vi "Analog Input.vi"() -> ()   [LabVIEW 2015]
doc: "Analog Input Example\n\nThis example will read voltages from an analog channel and display it on a chart. It will also display the average voltage over time. \n\nThe values for Average Bits and Samples Per Second on the front panel can be set while the VI is running.\n\nThis example expects a USB cable connected from your development PC to the Type B USB Jack (next to the power input) on the roboRIO."
uses:
  <vilib>/Rock Robotics/SystemInterfaces/AI/FPGA_AIChannel.ctl
  <vilib>/Rock Robotics/WPI/MotorControl/WPI_MotorControlDeviceRef.ctl
  <vilib>/Rock Robotics/WPI/MotorControl/WPI_MotorControlType.ctl
  <vilib>/Rock Robotics/SystemInterfaces/DIO/FPGA_DIOPWMChannel.ctl
  <vilib>/Rock Robotics/WPI/PWM/WPI_PWMDeadband.ctl
  <vilib>/Rock Robotics/WPI/CAN/Jaguar/SubVIs/WPI_CANJaguar_ControlMode.ctl
  <vilib>/Rock Robotics/WPI/CAN/TalonSRX/WPI_CANTalonSRX_APIControlMode.ctl
  <vilib>/Rock Robotics/WPI/MotorControl/WPI_MotorControlOpen Victor.vi
panel:
  out "MotorControlDevRef":T1={"DeviceStatus"={"status"=FALSE, "code"=0, "source"=""}, "Type"=enum."PWM", "PWM"={"PWM Channel"=enum."Invalid", "DeadBand"={"Name"="", "maxPositivePwm"=0, "minPositivePwm"=0, "centerPwm"=0, "maxNegativePwm"=0, "minNegativePwm"=0, "angularRange"=0}}, "CAN"={"Device Number"=0, "Control Mode"=enum."Percent VBus", "Semaphore"=refnum, "Max Vout"=12.0, "TalonSRX Control Mode"=enum."Percent VBus"}, "Invert"=FALSE}
  out "error out":errorcluster
  out "Motor Output":dbl
  in  "Output":dbl(slide) scale=-1.0..1.0
  in  "Samples Per Second":dbl=1000.0
  in  "Average Bits":u8=3 max=15
  in  "Channel":T8=enum."AI 2"
  out "Voltage Display":cluster{"Value":dbl, "Voltage":dbl}(graph)
  out "Average Voltage":dbl
  out "Voltage":dbl
  in  "stop":bool
  # "Set this input before running."
  # "These can be set while running."
  # "This chart displays the voltage and average voltage over time."
  # "This shows wiring for a typical analog input using a potentiometer.  In this case the potentiometer is being powered with 5 volts, and the Signal returned will vary from 0 to 5 volts"
  # "potentiometer"
  # "Gnd"
  # "S"
  # "V"
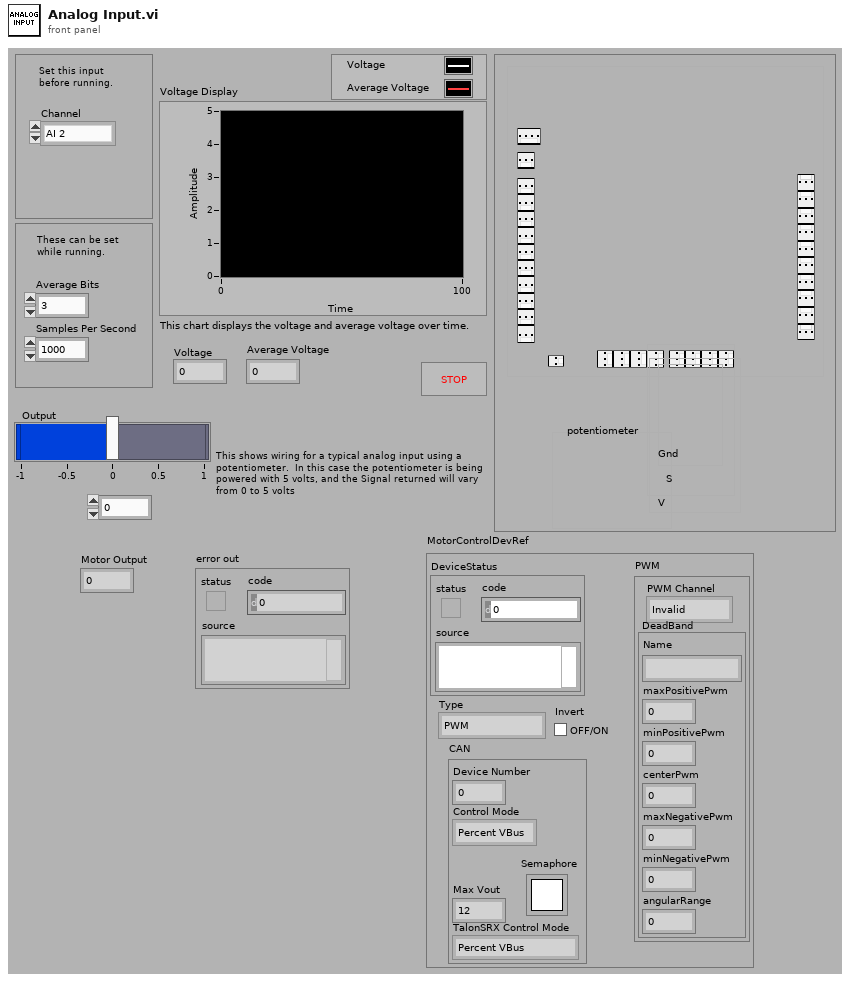
[diagram p1: front panel]
types:
  T1 = typedef "WPI_MotorControlDeviceRef.ctl" = cluster{"DeviceStatus":errorcluster, "Type":T2, "PWM":cluster{"PWM Channel":T3, "DeadBand":T4}, "CAN":cluster{"Device Number":u8, "Control Mode":T5, "Semaphore":T6, "Max Vout":dbl, "TalonSRX Control Mode":T7}, "Invert":bool}
  T2 = typedef "WPI_MotorControlType.ctl" = enum16{"PWM", "CAN", "CANTalonSRX"}
  T3 = typedef "FPGA_DIOPWMChannel.ctl" = enum8{"PWM 0", "PWM 1", "PWM 2", "PWM 3", "PWM 4", "PWM 5", "PWM 6", "PWM 7", "PWM 8", "PWM 9", "PWM MXP 0", "PWM MXP 1", "PWM MXP 2", "PWM MXP 3", "PWM MXP 4", "PWM MXP 5", "PWM MXP 6", "PWM MXP 7", "PWM MXP 8", "PWM MXP 9", "Invalid"}
  T4 = typedef "WPI_PWMDeadband.ctl" = cluster{"Name":string, "maxPositivePwm":i32, "minPositivePwm":i32, "centerPwm":i32, "maxNegativePwm":i32, "minNegativePwm":i32, "angularRange":u16}
  T5 = typedef "WPI_CANJaguar_ControlMode.ctl" = enum8{"Percent VBus", "Current", "Speed", "Position", "Voltage"}
  T6 = typedef "Semaphore RefNum" = refnum<k1>
  T7 = typedef "WPI_CANTalonSRX_APIControlMode.ctl" = enum8{"Percent VBus", "Speed", "Position", "Slave", "Unchanged / Invalid", "Voltage Compensation", "Current", "Motion Profile"}
  T8 = typedef "FPGA_AIChannel.ctl" = enum8{"AI 0", "AI 1", "AI 2", "AI 3", "AI MXP 0", "AI MXP 1", "AI MXP 2", "AI MXP 3", "Invalid"}
  T9 = typedef "WPI_AnalogChannelDevRef.ctl" = cluster{"DevStatus":errorcluster, "Analog Channel":T8}
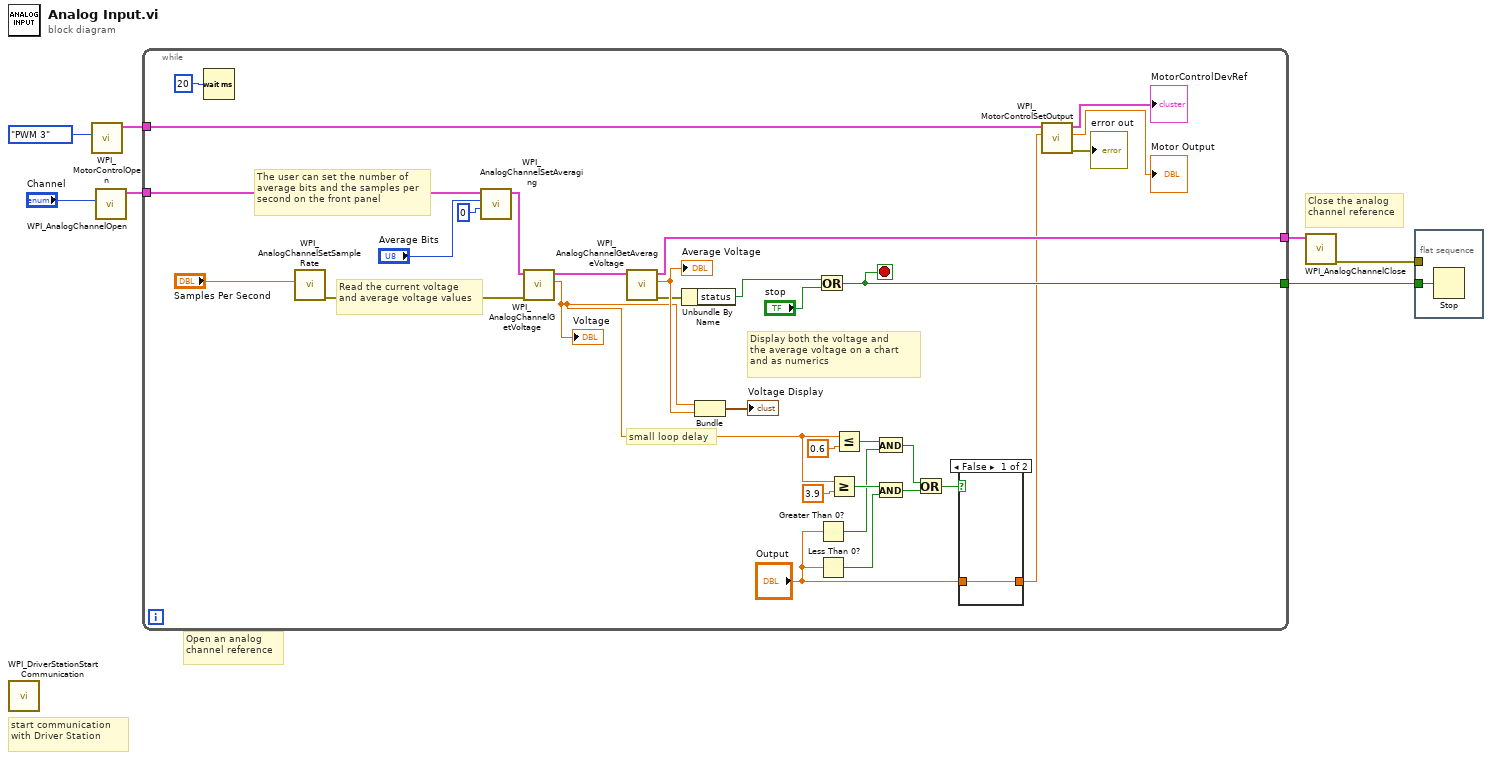
[diagram p0: block diagram]
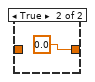
[diagram p2: hidden frame]
diagram:
  # "start communication with Driver Station"
  # "Close the analog\nchannel reference"
  # "Open an analog channel reference"
  n1 = call <vilib>:"WPI_DriverStationStart Communication.vi"() -> ()  [unwired: 2 in, 10 out]
  n2 = call-poly <vilib>:"WPI_MotorControlOpen.vi"("PWM Channel"=FPGA_DIOPWMChannel."PWM 3") -> ("MotorControlDeviceRef"=w1:T1)  [unwired: 9 in, 1 out]
  n3 = call <vilib>:"WPI_AnalogChannelOpen.vi"("Analog Channel"="Channel") -> ("AIDeviceRef"=w7:T9)  [unwired: 2 in, 8 out]
  n4 = while {
    tunnel: w7 -> [w33]
    tunnel: [w37] -> w6
    tunnel: [w24] -> w4
    tunnel: w1 -> [w23]
    stop <- w24 stop-if-true
    # "small loop delay"
    # "Read the current voltage\nand average voltage values"
    # "Display both the voltage and\nthe average voltage on a chart\nand as numerics"
    # "The user can set the number of \naverage bits and the samples per\nsecond on the front panel"
    n5 = Wait (ms)(milliseconds to wait=u32 20) -> ()  [unwired: 1 out]
    n6 = call <vilib>:"WPI_AnalogChannelSetSampleRate.vi"("Samples Per Second (per channel)"="Samples Per Second") -> ("error out"=w25:errorcluster)  [unwired: 4 in, 6 out]
    n7 = call <vilib>:"WPI_AnalogChannelSetAveraging.vi"("OversampleBits"=u8 0, "AverageBits"="Average Bits", "AIDeviceRef"=w33) -> ("AIDeviceRef"=w27:T9)  [unwired: 1 in, 7 out]
    n8 = call <vilib>:"WPI_AnalogChannelGetVoltage.vi"("error in (no error)"=w25, "AIDeviceRef"=w27) -> ("Voltage"=w12:dbl, "AIDeviceRef"=w38:T9)  [unwired: 8 out]
    "Voltage" <- w12
    n9 = call <vilib>:"WPI_AnalogChannelGetAverageVoltage.vi"("AIDeviceRef"=w38) -> ("error out"=w26:errorcluster, "Voltage"=w36:dbl, "AIDeviceRef"=w37:T9)  [unwired: 1 in, 7 out]
    "Average Voltage" <- w36
    n10 = Unbundle By Name(w26) -> ("status"=w31:bool)
    n11 = Bundle("Voltage"=w12, "Voltage"=w36) -> (→"Voltage Display":cluster{"Voltage":dbl, "Voltage":dbl})  [unwired: 1 out]
    n12 = Or(x=w31, y="stop") -> (x .or. y?=w24:bool)
    n13 = Greater Than 0?(x="Output") -> (x > 0?=w9:bool)
    n14 = Less Than 0?(x="Output") -> (x < 0?=w17:bool)
    n15 = Greater Or Equal?(x=w12, y=3.9) -> (x >= y?=w16:bool)
    n16 = Less Or Equal?(x=w12, y=0.6) -> (x <= y?=w11:bool)
    n17 = And(x=w11, y=w9) -> (x .and. y?=w8:bool)
    n18 = And(x=w16, y=w17) -> (x .and. y?=w15:bool)
    n19 = Or(x=w8, y=w15) -> (x .or. y?=w14:bool)
    n20 = case shown="False" w14 {
      tunnel: [w39 0.0] -> w22
      tunnel: "Output" -> [w39 _]
      frame False {
      }
      frame True {
      }
    }
    n21 = call <vilib>:"WPI_MotorControlSetOutput.vi"("Output"=w22, "MotorControlDevRef"=w23) -> ("error out"=→"error out":errorcluster, "Motor Output"=→"Motor Output":dbl, "MotorControlDevRef"=→"MotorControlDevRef":T1)  [unwired: 7 in]
  }
  n22 = call <vilib>:"WPI_AnalogChannelClose.vi"("AIDeviceRef"=w6) -> ("error out"=w3:errorcluster)  [unwired: 1 in, 9 out]
  n23 = flat-sequence {
    tunnel: w4 -> [w41]
    tunnel: w3 -> [_]
    frame #0 {
      n24 = Stop(stop? (T)=w41) -> ()
    }
  }
